vi "GetScale.vi"(11 "Properties":T1[](array[typedef])) -> (1 "offset":dbl, 3 "slope":dbl)   [LabVIEW 2017, in "ScanEngine.lvlib"]
uses:
  <vilib>/addons/InsightCM/Devices/Shared/Common/ScanEngine/ScanEngine.lvlib
  <vilib>/addons/InsightCM/MessageBus/Base/controls/KeyValuePair.ctl
  <vilib>/addons/InsightCM/Utilities/PropertyHelpers/PropertyHelpers.lvlib
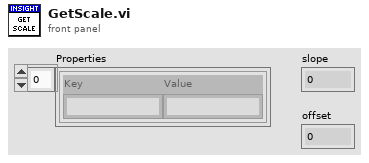
[diagram p1: front panel]
types:
  T1 = typedef "KeyValuePair.ctl" = cluster{"Key":string, "Value":string}
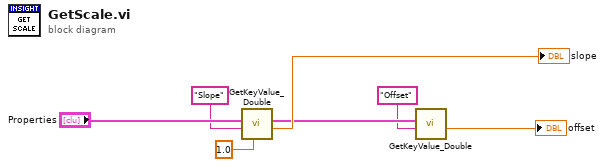
[diagram p0: block diagram]
diagram:
  n1 = call <vilib>:"GetKeyValue_Double.vi"("default"=1.0, "key"="Slope", "key value pairs"="Properties") -> ("value"=→"slope":dbl, "key value pairs out"=w4:T1[])  [unwired: 6 in, 1 out]
  n2 = call <vilib>:"GetKeyValue_Double.vi"("key"="Offset", "key value pairs"=w4) -> ("value"=→"offset":dbl)  [unwired: 7 in, 2 out]
